vi "checkForceP.vi"(8 "error in (no error)":errorcluster, 11 "Model in":refnum<class "Model.lvclass">) -> (0 "error out":errorcluster, 2 "reachedForceTriggerIsTrue":bool, 3 "Model out":refnum<class "Model.lvclass">)   [LabVIEW 2015, in "Model.lvclass"]
uses:
  Model.lvclass
  Model.lvclass/Model.ctl
  <userlib>/Common/Devices/ForceSensorCalculator/ForceSensorCalculator/ForceSensorCalculator.lvclass/ForceSensorCalculator.ctl
  <userlib>/Common/Devices/ForceSensorCalculator/ForceSensorCalculator/ForceSensorCalculator.lvclass
  ApplicationElements/SystemController/SystemController.lvclass
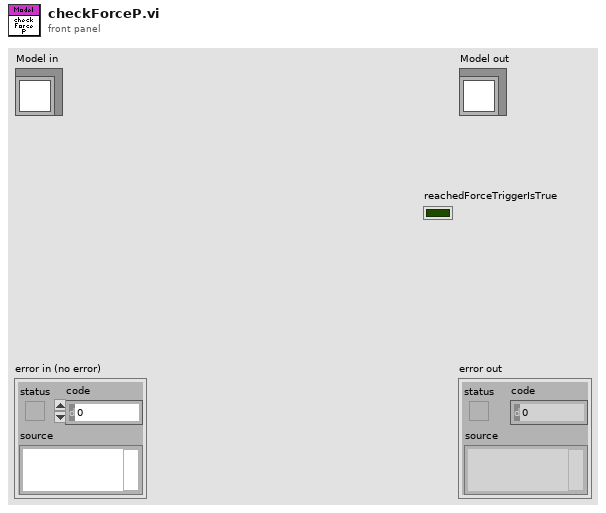
[diagram p1: front panel]
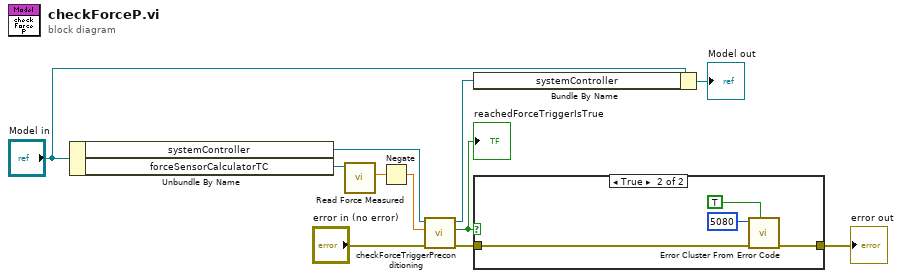
[diagram p0: block diagram]
diagram:
  n1 = Unbundle By Name("Model in") -> ("systemController"=w9:refnum<class "SystemController.lvclass">, "forceSensorCalculatorTC"=w6:refnum<class "ForceSensorCalculatorTC.lvclass">)
  n2 = call <userlib>:"Read Force Measured.vi"("ForceSensor in"=w6) -> ("Force Demand"=w5:dbl[unit])  [unwired: 9 in, 1 out]
  n3 = Negate(x=w5) -> (-x=w1:dbl[unit])
  n4 = call "checkForceTriggerPreconditioning.vi"("error in (no error)"="error in (no error)", "Force Measured"=w1, "SystemController in"=w9) -> ("error out"=w4:errorcluster, "forceTriggerReached"=w2:bool, "SystemController out"=w8:refnum<class "SystemController.lvclass">)  [unwired: 6 in]
  "reachedForceTriggerIsTrue" <- w2
  n5 = Bundle By Name(cluster="Model in", "systemController"=w8) -> (→"Model out":refnum<class "Model.lvclass">)
  n6 = case shown="True" w2 {
    tunnel: w4 -> [w12 w15]
    tunnel: [w12 w14] -> w3
    frame False {
    }
    frame True {
      n7 = call <vilib>:"Error Cluster From Error Code.vi"("show call chain? (False)"=TRUE, "error in (no error)"=w15, "error code (0)"=5080) -> ("error out"=w14:errorcluster)  [unwired: 6 in]
    }
  }
  "error out" <- w3
